vi "Process Handler State(End Spawn Processes).vi"(0 "Process Handler In":refnum<class "Process Handler.lvclass">, 1 "Process Variables In":T1, 11 "Error In":errorcluster) -> (3 "Process Variables Out":T1, 4 "Process Handler Out":refnum<class "Process Handler.lvclass">, 15 "Error Out":errorcluster)   [LabVIEW 2023, in "Process Handler.lvclass"]
doc: "Method encapsulating End Spawn Processes state of Process Handler.\n\nSends information about number of spawn processes to Clean Up method, then stops all spawn processes one by one, and sends confirmation."
uses:
  Process Handler.lvclass
  Private/Ctrls/Process Variables.ctl
  Process/Process.lvclass
  Interfaces/ICanCommunicate/Message.ctl
  Process Handler.lvclass/Process Handler.ctl
  Interfaces/ICanCommunicate/ICanCommunicate.lvclass
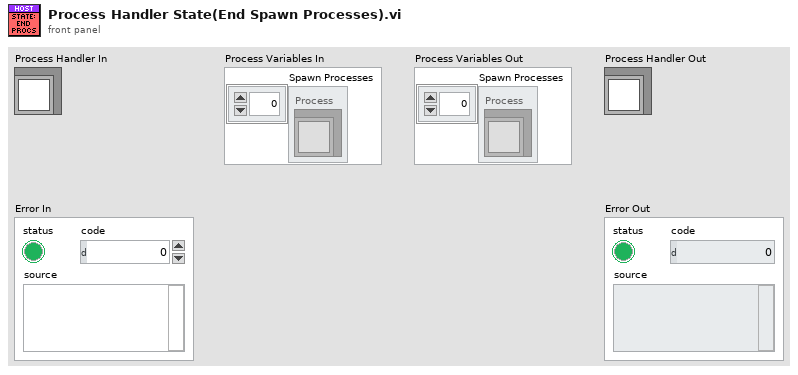
[diagram p1: front panel]
types:
  T1 = typedef "Process Handler.lvclass/Process Variables.ctl" = cluster{"Spawn Processes":refnum<class "Process.lvclass">[]}
  T2 = typedef "ICanCommunicate.lvclass/ProcessSyncQueue.ctl" = refnum<queue>
  T3 = typedef "ICanCommunicate.lvclass/FromProcessQueue.ctl" = refnum<queue>
  T4 = typedef "ICanCommunicate.lvclass/Message.ctl" = cluster{"Sender Name":string, "Recipent Name":string, "Command":string, "Data":variant, "Time Stamp":timestamp, "GUID":string, "Chcecksum":string}
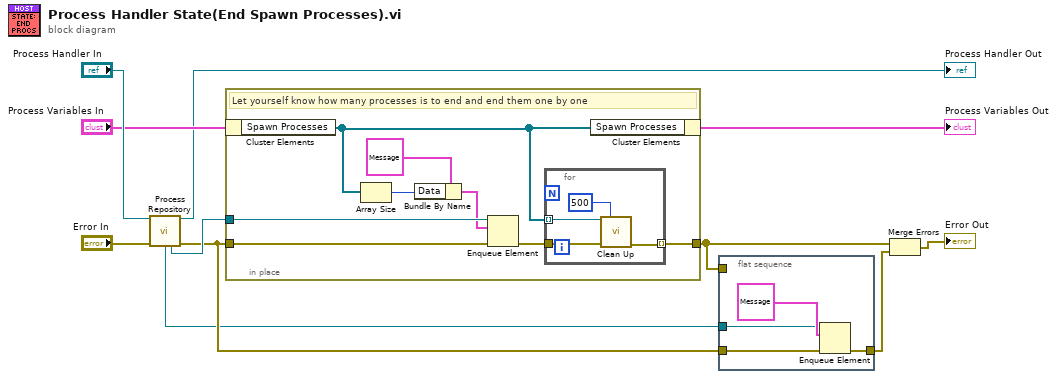
[diagram p0: block diagram]
diagram:
  n1 = call-dynamic "Process Repository.vi"("Process In"="Process Handler In", "Error In"="Error In") -> ("Process Out"=→"Process Handler Out":refnum<class "Process Handler.lvclass">, "ProcessSyncQueue"=w8:T2, "FromProcessQueue"=w11:T3, "Error Out"=w10:errorcluster)  [unwired: 7 in, 3 out]
  n2 = in-place {
    in-place-border: w10 -> [w19]
    in-place-border: [w18] -> w6
    in-place-border: w11 -> [w15]
    # "Let yourself know how many processes is to end and end them one by one"
    n3 = in-place-cluster #1("Process Variables In") -> ("Spawn Processes"=w17:refnum<class "Process.lvclass">[])
    n4 = Array Size(array=w17) -> (size(s)=w13:i32)
    n5 = Bundle By Name(cluster=T4 {"Sender Name"="", "Recipent Name"="", "Command"="Spawn Processes", "Data"=variant, "Time Stamp"=timestamp(0 s since 1904-01-01), "GUID"="", "Chcecksum"=""} ("element"), "Data"=w13) -> (w12:T4)
    n6 = Enqueue Element(queue=w15, element=w12, error in (no error)=w19) -> (error out=w16:errorcluster)  [unwired: 1 in, 2 out]
    n7 = for {
      tunnel: w17 -> [w21] mode=indexing
      tunnel: w16 -> [w23]
      tunnel: [w22] -> w18 mode=indexing
      n8 = call-dynamic "Clean Up.vi"("Process In"=w21, "Timeout in ms (-1)"=500, "Error In"=w23) -> ("Error Out"=w22:errorcluster)  [unwired: 11 in, 1 out]
    }
    n9 = in-place-cluster #1("Spawn Processes"=w17) -> (→"Process Variables Out":T1)
  }
  n10 = flat-sequence {
    tunnel: [w27] -> w5
    tunnel: w6 -> [_]
    tunnel: w8 -> [w25]
    tunnel: w10 -> [w24]
    frame #0 {
      n11 = Enqueue Element(queue=w25, element=T4 {"Sender Name"="", "Recipent Name"="", "Command"="Close", "Data"=variant, "Time Stamp"=timestamp(0 s since 1904-01-01), "GUID"="", "Chcecksum"=""}, error in (no error)=w24) -> (error out=w27:errorcluster)  [unwired: 1 in, 2 out]
    }
  }
  n12 = Merge Errors(w6, w5) -> (→"Error Out":errorcluster)
